vi "Utilities_Read_Files.vi"() -> ()   [LabVIEW 2020]
panel:
  out "data":string[](array[string])
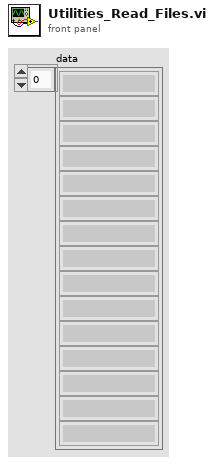
[diagram p1: front panel]
types:
  T1 = enum16{"open", "open or create", "create or replace", "create", "open (read-only)"}
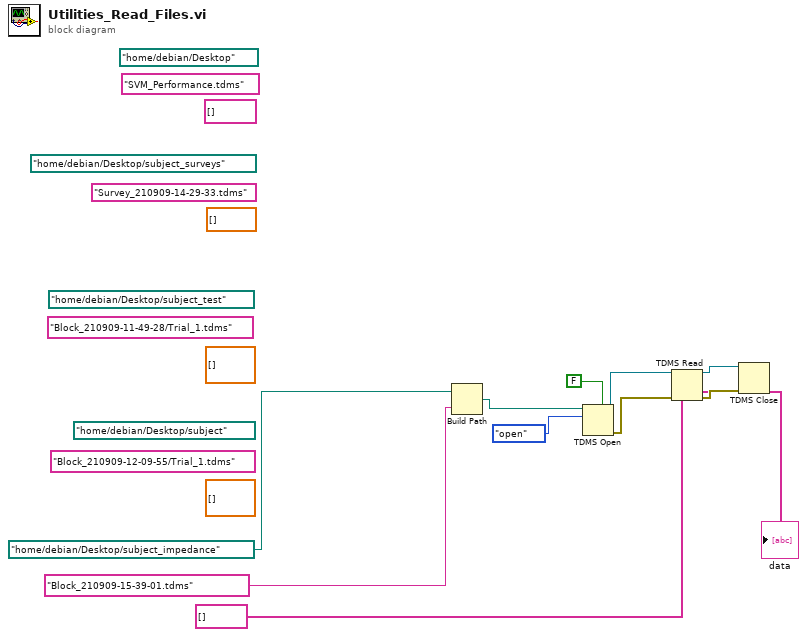
[diagram p0: block diagram]
diagram:
  (unwired) "Block_210909-12-09-55/Trial_1.tdms"
  (unwired) dbl[][] []
  (unwired) string[] []
  (unwired) "SVM_Performance.tdms"
  (unwired) dbl[][] []
  (unwired) "Block_210909-11-49-28/Trial_1.tdms"
  (unwired) dbl[] []
  (unwired) "Survey_210909-14-29-33.tdms"
  (unwired) path "/home/debian/Desktop" ("base path")
  (unwired) path "/home/debian/Desktop/subject" ("base path")
  (unwired) path "/home/debian/Desktop/subject_test" ("base path")
  (unwired) path "/home/debian/Desktop/subject_surveys" ("base path")
  n1 = Build Path(base path=path "/home/debian/Desktop/subject_impedance", name or relative path="Block_210909-15-39-01.tdms") -> (appended path=w11:path)
  n2 = TDMS Open(5:FALSE ("create index file? (T)"), 10:T1."open" ("operation (0:open)"), 11:w11) -> (0:w9:errorcluster, 3:w7:refnum<k34>)  [unwired: 4 in]
  n3 = TDMS Read(0:w7, 11:w9, 12:string[] []) -> (4:w6:refnum<k34>, 10:→"data":string[], 15:w8:errorcluster)  [unwired: 5 in, 3 out]
  n4 = TDMS Close(8:w8, 11:w6) -> ()  [unwired: 2 out]
